vi "convertRampAttributesStringToLVData.vi"(8 "error in (no error)":errorcluster, 11 "Job Ramp Array":string[](array[string])) -> (0 "error out":errorcluster, 2 "Duration":dbl, 3 "Setpoint":u16)   [LabVIEW 2021]
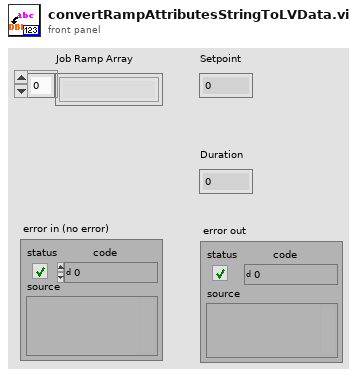
[diagram p1: front panel]
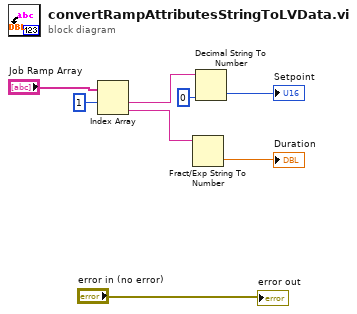
[diagram p0: block diagram]
diagram:
  n1 = Index Array(array="Job Ramp Array", index #1=1 ("index")) -> (element #1=w5:string, element #2=w7:string)  [unwired: 1 in]
  n2 = Fract/Exp String To Number(string=w7) -> (number=→"Duration":dbl)  [unwired: 3 in, 1 out]
  n3 = Decimal String To Number(string=w5, default (0L)=u16 0 ("default (0 I32)")) -> (number=→"Setpoint":u16)  [unwired: 1 in, 1 out]
  "error out" <- "error in (no error)"
